vi "INBETRIEBNAHME SONIMIX 2106-LCD.vi"() -> ()   [LabVIEW 2015, in "Linearisierung v2.lvlib" / "Gasteiler.lvlib" / "AK Komm Gasteiler.lvlib"]
uses:
  AK Komm Gasteiler.lvlib
  AK-Schnittstelle/Seriell - Baud Rate.ctl
  AK-Schnittstelle/AK Seriell/AK Seriell.lvlib
  AK-Schnittstelle/Seriell - Data Bits.ctl
  AK-Schnittstelle/Seriell - Flow Control.ctl
  AK-Schnittstelle/Seriell - Parity Bits.ctl
  AK-Schnittstelle/Seriell - Stop Bits.ctl
  Visualisierungs Elemente/VISA Control.ctl
panel:
  in  "löschen":bool
  out "Daten":string
  in  "Schnittstelle":T7={"VISA Resource Name"="COM1", "Baud Rate"=9600, "data bits"=8, "parity"=0, "stop bits"=10, "flow control"=0} {"stop bits" items=["1.0"=10, "1.5"=15, "2.0"=20]; "parity" items=["None", "Odd", "Even", "Mark", "Space"]; "flow control" items=["None"=0, "XON/XOFF"=1, "RTS/CTS"=2, "DTR/DSR"=4]; "data bits" items=["8"=8, "7"=7, "6"=6, "5"=5, "4"=4]; "Baud Rate" items=["38400"=38400, "19200"=19200, "14400"=14400, "9600"=9600, "4800"=4800, "2400"=2400]}
  out "Befehl (Antwort)":string
  in  "TimeOut (ms)":u32=10000
  out "Empfangsdaten":string[](array[string])
  out "ES (Error Status)":string
  in  "Sendedaten":string[](array[string])
  in  "Kanalnummer (0)":u8
  in  "Befehl (4 Zeichen)":string="STBY"
  out "error out":errorcluster caption="Fehler (Ausgang)"
  in  "ausführen":bool
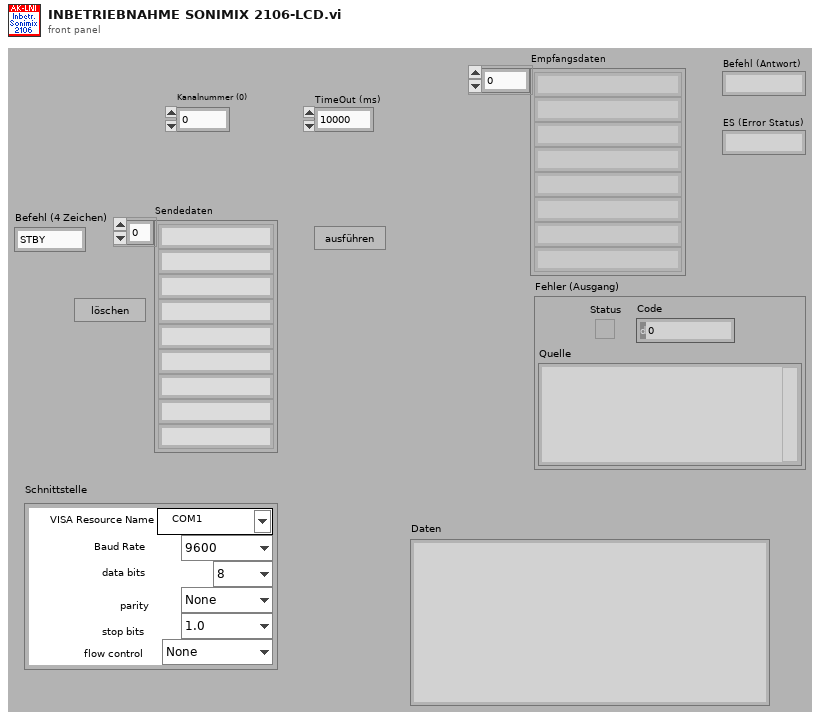
[diagram p1: front panel]
types:
  T1 = typedef "VISA Control.ctl" = refnum<visa-resource-name>
  T2 = typedef "AK-Schnittstelle.lvlib/AK Seriell.lvlib/Seriell - Baud Rate.ctl" = u16
  T3 = typedef "AK-Schnittstelle.lvlib/AK Seriell.lvlib/Seriell - Data Bits.ctl" = u16
  T4 = typedef "AK-Schnittstelle.lvlib/AK Seriell.lvlib/Seriell - Parity Bits.ctl" = u16
  T5 = typedef "AK-Schnittstelle.lvlib/AK Seriell.lvlib/Seriell - Stop Bits.ctl" = u16
  T6 = typedef "AK-Schnittstelle.lvlib/AK Seriell.lvlib/Seriell - Flow Control.ctl" = u16
  T7 = cluster{"VISA Resource Name":T1, "Baud Rate":T2, "data bits":T3, "parity":T4, "stop bits":T5, "flow control":T6}
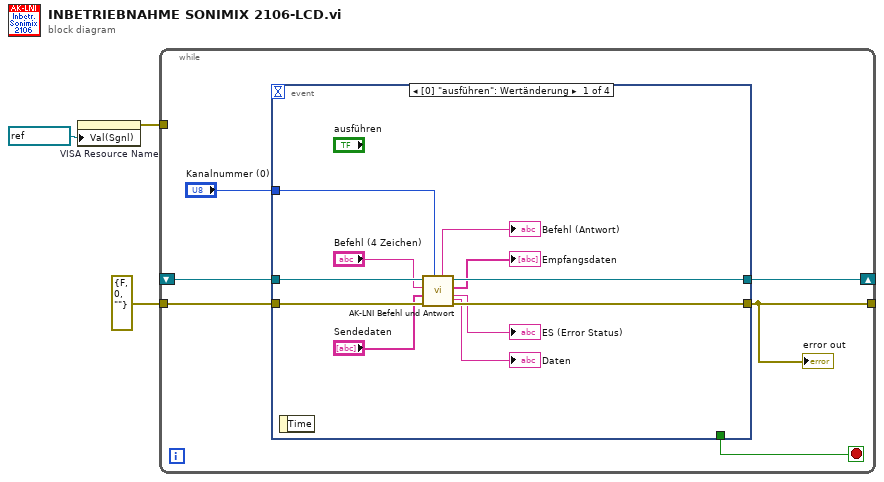
[diagram p0: block diagram]
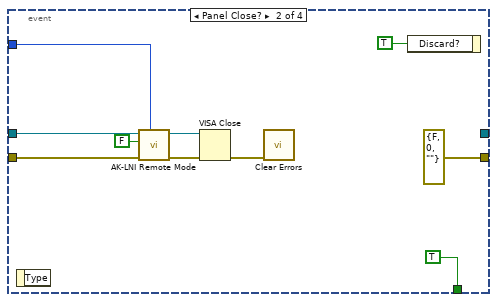
[diagram p2: hidden frame]
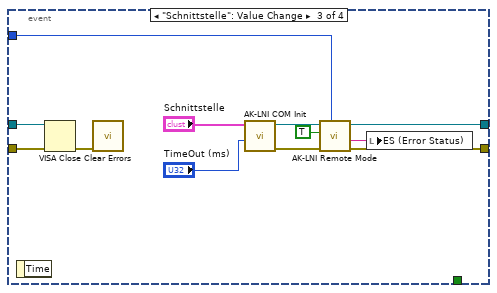
[diagram p3: hidden frame]
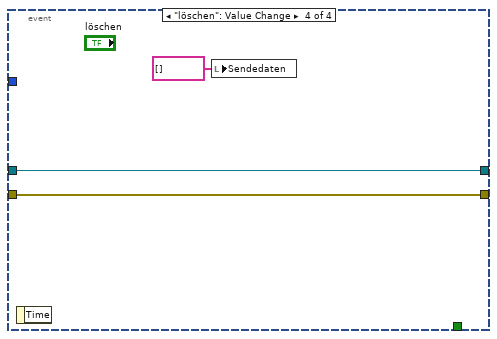
[diagram p4: hidden frame]
diagram:
  n1 = property on="VISA Resource Name" class="VISAName (strikt)"("Val(Sgnl)"=refnum<visa-resource-name> "COM1" ("Wert (signalisierend)")) -> (error out=w3:errorcluster)  [unwired: 2 in, 1 out]
  n2 = while {
    shift-right: [w7] -> _
    shift-left: _ -> [w9]
    tunnel: w3 -> [_]
    tunnel: errorcluster {"status"=FALSE, "code"=0, "source"=""} ("Fehler (Eingang, kein Fehler)") -> [w8]
    tunnel: [w4] -> _
    stop <- w6 stop-if-true
    n3 = event shown="[0] \"ausführen\": Wertänderung" {
      selector: _ -> [_ _ _ _]
      dyn-events: _ -> [_ _ _ _]
      timeout: _ -> [_ _ _ _]
      tunnel: w9 -> [w20 w27 w42 w45]
      tunnel: w8 -> [w19 w25 w41 w44]
      tunnel: [w18 _ w38 w45] -> w7
      tunnel: [w17 errorcluster {"status"=FALSE, "code"=0, "source"=""} ("Fehler (Ausgang)") w36 w44] -> w4
      tunnel: [_ TRUE _ _] -> w6
      tunnel: "Kanalnummer (0)" -> [w15 w22 w34 _]
      event "ausführen": Value Change {
        n4 = event-data() -> ()  [unwired: 1 in, 1 out]
        n5 = call "AK-LNI Befehl und Antwort.vi"("Kanalnummer (0)"=w15, "Fehler (Eingang)"=w19, "Sendedaten"="Sendedaten", "Befehl (4 Zeichen)"="Befehl (4 Zeichen)", "VISA resource name"=w20) -> ("Fehler (Ausgang)"=w17:errorcluster, "ES (Error Status)"=→"ES (Error Status)":string, "Empfangsdaten"=→"Empfangsdaten":string[], "VISA resource name out"=w18:refnum<visa-resource-name>, "Daten"=→"Daten":string, "Befehl (Antwort)"=→"Befehl (Antwort)":string)  [unwired: 1 in]
      }
      event Panel Close? {
        n6 = event-data() -> ()  [unwired: 1 in, 1 out]
        n7 = call "AK-LNI Remote Mode.vi"("Kanalnummer (K0)"=w22, "Fehler (Eingang)"=w25, "Remote"=FALSE ("remote"), "VISA resource name"=w27) -> ("Fehler (Ausgang)"=w24:errorcluster, "VISA resource name out"=w26:refnum<visa-resource-name>)  [unwired: 5 in, 1 out]
        n8 = VISA Close(VISA resource name=w26, error in (no error)=w24) -> (error out=w29:errorcluster)
        n9 = call <vilib>:"Clear Errors.vi"("error in (no error)"=w29) -> ()  [unwired: 5 in, 2 out]
        n10 = event-data("Discard?"=TRUE ("Verwerfen?")) -> ()  [unwired: 1 in, 1 out]
      }
      event "Schnittstelle": Value Change {
        n11 = event-data() -> ()  [unwired: 1 in, 1 out]
        n12 = VISA Close(VISA resource name=w42, error in (no error)=w41) -> (error out=w40:errorcluster)
        n13 = call <vilib>:"Clear Errors.vi"("error in (no error)"=w40) -> ()  [unwired: 5 in, 2 out]
        n14 = call "AK-LNI COM Init.vi"("TimeOut (ms)"="TimeOut (ms)", "Schnittstelle"="Schnittstelle") -> ("error out"=w37:errorcluster, "VISA resource name"=w39:refnum<visa-resource-name>)  [unwired: 8 in]
        n15 = call "AK-LNI Remote Mode.vi"("Kanalnummer (K0)"=w34, "Fehler (Eingang)"=w37, "Remote"=TRUE ("remote"), "VISA resource name"=w39) -> ("Fehler (Ausgang)"=w36:errorcluster, "ES (Error Status)"=w32:string, "VISA resource name out"=w38:refnum<visa-resource-name>)  [unwired: 5 in]
        n16 = local write "ES (Error Status)"(w32) -> ()
      }
      event "löschen": Value Change {
        n17 = event-data() -> ()  [unwired: 1 in, 1 out]
        n18 = local write "Sendedaten"(string[] [] ("Sendedaten")) -> ()
      }
    }
    "error out" <- w4
  }
